vi "DIO fpga.vi"(10 "I/O项":bool, 11 "引用句柄输入":refnum<k21>) -> ()   [LabVIEW 2017]
uses:
  <vilib>/rvi/eio/common/nirviEmuTemplateMethod_errors.vi
  <vilib>/eio/EIOMethodNode/EIOMethodNode.xnode
  <vilib>/eio/EIONode/EIONode.xnode
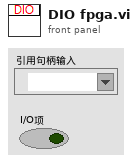
[diagram p1: front panel]
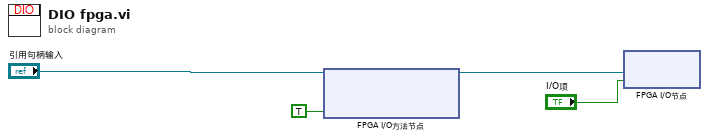
[diagram p0: block diagram]
diagram:
  n1 = xnode "FPGA I/O方法节点"("FPGA I/O In"="引用句柄输入", "Enable"=TRUE) -> ("FPGA I/O Out"=w1:refnum<k21>)
  n2 = xnode "FPGA I/O节点"("I/O项"="I/O项", "FPGA I/O输入"=w1) -> ()  [unwired: 1 out]
